vi "Lab Panel V4.86.vi"() -> ()   [LabVIEW 2013] (continued)
                  tunnel: w5309 -> [w5337 w5340]
                  tunnel: [w5337 w5339] -> w5307
                  frame False {
                  }
                  frame True {
                    n2929 = Multiply(x=w5341, y=w5340) -> (x*y=w5339:dbl)
                    n2930 = Multiply(x=w5341, y=w5343) -> (x*y=w5342:dbl)
                  }
                }
                n2931 = local read "SIG LAB05-1"() -> (w5328:T2)
                n2932 = Bundle By Name(cluster=w5328, "Tmp Live"=w5308, "Tmp Neut"=w5307) -> (w5327:T2)
                n2933 = local read "SIG LAB05-2"() -> (w5326:T2)
                n2934 = Bundle By Name(cluster=w5326, "Tmp Live"=w5304, "Tmp Neut"=w5303) -> (w5325:T2)
                n2935 = local write "SIG LAB05-1"(w5327) -> ()
                n2936 = local write "SIG LAB05-2"(w5325) -> ()
              }
            }
          }
          frame #20 {
            # "write data to display panel"
            n2937 = global write "Global display 1.vi" "TEST 5-2"(w5380) -> ()
            n2938 = global write "Global display 1.vi" "TEST 4-2"(w5382) -> ()
            n2939 = global write "Global display 1.vi" "TEST 1-2"(w5388) -> ()
            n2940 = global write "Global display 1.vi" "TEST 3-1"(w5385) -> ()
            n2941 = global write "Global display 1.vi" "TEST 5-1"(w5381) -> ()
            n2942 = global write "Global display 1.vi" "TEST 1-1"(w5389) -> ()
            n2943 = global write "Global display 1.vi" "TEST 3-2"(w5384) -> ()
            n2944 = global write "Global display 1.vi" "TEST 4-1"(w5383) -> ()
            n2945 = global write "Global display 1.vi" "TEST 2-2"(w5386) -> ()
            n2946 = global write "Global display 1.vi" "TEST 2-1"(w5387) -> ()
            n2947 = global read "Global display 3.vi" "log 1-1"() -> (→"LOG LAB01-1":string)
            n2948 = global read "Global display 3.vi" "log 3-1"() -> (→"LOG LAB03-1":string)
            n2949 = global read "Global display 3.vi" "log 1-2"() -> (→"LOG LAB01-2":string)
            n2950 = property on="Tab Control 2" class="TabCtl (strict)"() -> ("Pages"=w5379:refnum<vi>[])  [unwired: 2 in, 2 out]
            n2951 = global read "Global display 3.vi" "log 2-1"() -> (→"LOG LAB02-1":string)
            n2952 = global read "Global display 3.vi" "log 2-2"() -> (→"LOG LAB02-2":string)
            n2953 = global read "Global display 3.vi" "log 4-2"() -> (→"LOG LAB04-2":string)
            n2954 = global read "Global display 3.vi" "log 5-2"() -> (→"LOG LAB05-2":string)
            n2955 = global read "Global display 3.vi" "log 5-1"() -> (→"LOG LAB05-1":string)
            n2956 = global read "Global display 3.vi" "log 4-1"() -> (→"LOG LAB04-1":string)
            n2957 = global read "Global display 3.vi" "log 3-2"() -> (→"LOG LAB03-2":string)
            n2958 = Index Array(array=w5379, index=9) -> (element=w5377:refnum<vi>)
            n2959 = property class="Page"(reference=w5377) -> ("PageVis"=w5376:bool)  [unwired: 1 in, 2 out]
            n2960 = global write "Global display 3.vi" "admin"(w5376) -> ()
            n2961 = local read "O/I  LAB05-2"() -> (w5430:bool)
            n2962 = local read "O/I  LAB05-1"() -> (w5431:bool)
            n2963 = local read "O/I  LAB03-2"() -> (w5434:bool)
            n2964 = local read "O/I  LAB04-2"() -> (w5432:bool)
            n2965 = local read "O/I  LAB04-1"() -> (w5433:bool)
            n2966 = local read "O/I  LAB03-1"() -> (w5435:bool)
            n2967 = local read "O/I  LAB01-2"() -> (w5438:bool)
            n2968 = local read "O/I  LAB01-1"() -> (w5439:bool)
            n2969 = local read "O/I  LAB02-1"() -> (w5437:bool)
            n2970 = local read "O/I  LAB02-2"() -> (w5436:bool)
            n2971 = global write "Global display 1.vi" "5-2 O/F"(w5430) -> ()
            n2972 = global write "Global display 1.vi" "5-1 O/F"(w5431) -> ()
            n2973 = global write "Global display 1.vi" "4-1 O/F"(w5433) -> ()
            n2974 = global write "Global display 1.vi" "4-2 O/F"(w5432) -> ()
            n2975 = global write "Global display 1.vi" "3-2 O/F"(w5434) -> ()
            n2976 = global write "Global display 1.vi" "3-1 O/F"(w5435) -> ()
            n2977 = global write "Global display 1.vi" "2-2 O/F"(w5436) -> ()
            n2978 = global write "Global display 1.vi" "2-1 O/F"(w5437) -> ()
            n2979 = global write "Global display 1.vi" "1-2 O/F"(w5438) -> ()
            n2980 = global write "Global display 1.vi" "1-1 O/F"(w5439) -> ()
            n2981 = local read "TEMP START LAB02-2"() -> (w5362:cluster{"TL":dbl, "TN":dbl})
            n2982 = local read "run lab05-2"() -> (w5420:bool)
            n2983 = local read "TEMP START LAB01-2"() -> (w5364:cluster{"TL":dbl, "TN":dbl})
            n2984 = local read "TEMP START LAB02-1"() -> (w5363:cluster{"TL":dbl, "TN":dbl})
            n2985 = local read "TEMP START LAB04-1"() -> (w5359:cluster{"TL":dbl, "TN":dbl})
            n2986 = local read "TEMP START LAB04-2"() -> (w5358:cluster{"TL":dbl, "TN":dbl})
            n2987 = local read "run lab04-1"() -> (w5423:bool)
            n2988 = local read "run lab04-2"() -> (w5422:bool)
            n2989 = local read "run lab05-1"() -> (w5421:bool)
            n2990 = local read "TEMP START LAB01-1"() -> (w5365:cluster{"TL":dbl, "TN":dbl})
            n2991 = local read "TEMP START LAB05-2"() -> (w5356:cluster{"TL":dbl, "TN":dbl})
            n2992 = local read "TEMP START LAB05-1"() -> (w5357:cluster{"TL":dbl, "TN":dbl})
            n2993 = local read "run lab03-2"() -> (w5424:bool)
            n2994 = local read "TEMP START LAB03-2"() -> (w5360:cluster{"TL":dbl, "TN":dbl})
            n2995 = local read "TEMP START LAB03-1"() -> (w5361:cluster{"TL":dbl, "TN":dbl})
            n2996 = local read "run lab02-1"() -> (w5427:bool)
            n2997 = local read "run lab03-1"() -> (w5425:bool)
            n2998 = local read "run lab01-2"() -> (w5428:bool)
            n2999 = local read "run lab02-2"() -> (w5426:bool)
            n3000 = local read "run lab01-1"() -> (w5429:bool)
            n3001 = global write "Global display 1.vi" "5-2 R/S"(w5420) -> ()
            n3002 = global write "Global display 1.vi" "5-1 R/S"(w5421) -> ()
            n3003 = global write "Global display 1.vi" "4-2 R/S"(w5422) -> ()
            n3004 = global write "Global display 1.vi" "4-1 R/S"(w5423) -> ()
            n3005 = global write "Global display 1.vi" "3-2 R/S"(w5424) -> ()
            n3006 = global write "Global display 1.vi" "1-2 R/S"(w5428) -> ()
            n3007 = global write "Global display 1.vi" "2-1 R/S"(w5427) -> ()
            n3008 = global write "Global display 1.vi" "3-1 R/S"(w5425) -> ()
            n3009 = global write "Global display 1.vi" "2-2 R/S"(w5426) -> ()
            n3010 = global write "Global display 1.vi" "1-1 R/S"(w5429) -> ()
            n3011 = global write "Global display 3.vi" "TEMP ST 05-2"(w5356) -> ()
            n3012 = global write "Global display 3.vi" "TEMP ST 05-1"(w5357) -> ()
            n3013 = global write "Global display 3.vi" "TEMP ST 03-2"(w5360) -> ()
            n3014 = global write "Global display 3.vi" "TEMP ST 04-2"(w5358) -> ()
            n3015 = global write "Global display 3.vi" "TEMP ST 01-1"(w5365) -> ()
            n3016 = global write "Global display 3.vi" "TEMP ST 01-2"(w5364) -> ()
            n3017 = global write "Global display 3.vi" "TEMP ST 04-1"(w5359) -> ()
            n3018 = global write "Global display 3.vi" "TEMP ST 02-1"(w5363) -> ()
            n3019 = global write "Global display 3.vi" "TEMP ST 02-2"(w5362) -> ()
            n3020 = global write "Global display 3.vi" "TEMP ST 03-1"(w5361) -> ()
            n3021 = local read "DISP LAB04-2"() -> (w5412:T4)
            n3022 = local read "DISP LAB05-1"() -> (w5411:T4)
            n3023 = local read "DISP LAB04-1"() -> (w5413:T4)
            n3024 = local read "DISP LAB05-2"() -> (w5410:T4)
            n3025 = local read "DISP LAB03-1"() -> (w5415:T4)
            n3026 = local read "DISP LAB03-2"() -> (w5414:T4)
            n3027 = local read "DISP LAB01-2"() -> (w5418:T4)
            n3028 = local read "DISP LAB02-1"() -> (w5417:T4)
            n3029 = local read "DISP LAB02-2"() -> (w5416:T4)
            n3030 = local read "DISP LAB01-1"() -> (w5419:T4)
            n3031 = local read "TEMP RISE LAB05-1"() -> (w5347:cluster{"TL":dbl, "TN":dbl})
            n3032 = local read "TEMP RISE LAB05-2"() -> (w5346:cluster{"TL":dbl, "TN":dbl})
            n3033 = local read "TEMP RISE LAB04-2"() -> (w5348:cluster{"TL":dbl, "TN":dbl})
            n3034 = local read "TEMP RISE LAB04-1"() -> (w5349:cluster{"TL":dbl, "TN":dbl})
            n3035 = local read "TEMP RISE LAB03-2"() -> (w5350:cluster{"TL":dbl, "TN":dbl})
            n3036 = local read "TEMP RISE LAB03-1"() -> (w5351:cluster{"TL":dbl, "TN":dbl})
            n3037 = local read "TEMP RISE LAB01-2"() -> (w5354:cluster{"TL":dbl, "TN":dbl})
            n3038 = local read "TEMP RISE LAB02-2"() -> (w5352:cluster{"TL":dbl, "TN":dbl})
            n3039 = local read "TEMP RISE LAB01-1"() -> (w5355:cluster{"TL":dbl, "TN":dbl})
            n3040 = local read "TEMP RISE LAB02-1"() -> (w5353:cluster{"TL":dbl, "TN":dbl})
            n3041 = global write "Global display 2.vi" "DISP LAB05-1"(w5411) -> ()
            n3042 = global write "Global display 2.vi" "DISP LAB05-2"(w5410) -> ()
            n3043 = global write "Global display 2.vi" "DISP LAB04-2"(w5412) -> ()
            n3044 = global write "Global display 2.vi" "DISP LAB02-1"(w5417) -> ()
            n3045 = global write "Global display 2.vi" "DISP LAB02-2"(w5416) -> ()
            n3046 = global write "Global display 2.vi" "DISP LAB04-1"(w5413) -> ()
            n3047 = global write "Global display 2.vi" "DISP LAB01-2"(w5418) -> ()
            n3048 = global write "Global display 2.vi" "DISP LAB01-1"(w5419) -> ()
            n3049 = global write "Global display 2.vi" "DISP LAB03-1"(w5415) -> ()
            n3050 = global write "Global display 2.vi" "DISP LAB03-2"(w5414) -> ()
            n3051 = global write "Global display 3.vi" "TEMP RS 05-2"(w5346) -> ()
            n3052 = global write "Global display 3.vi" "TEMP RS 05-1"(w5347) -> ()
            n3053 = global write "Global display 3.vi" "TEMP RS 03-2"(w5350) -> ()
            n3054 = global write "Global display 3.vi" "TEMP RS 02-1"(w5353) -> ()
            n3055 = global write "Global display 3.vi" "TEMP RS 02-2"(w5352) -> ()
            n3056 = global write "Global display 3.vi" "TEMP RS 04-2"(w5348) -> ()
            n3057 = global write "Global display 3.vi" "TEMP RS 01-2"(w5354) -> ()
            n3058 = global write "Global display 3.vi" "TEMP RS 03-1"(w5351) -> ()
            n3059 = global write "Global display 3.vi" "TEMP RS 04-1"(w5349) -> ()
            n3060 = global write "Global display 3.vi" "TEMP RS 01-1"(w5355) -> ()
            n3061 = local read "SET LAB05-2"() -> (w5400:T5)
            n3062 = local read "SET LAB05-1"() -> (w5401:T5)
            n3063 = local read "SET LAB04-1"() -> (w5403:T5)
            n3064 = local read "SET LAB04-2"() -> (w5402:T5)
            n3065 = local read "SET LAB03-1"() -> (w5405:T5)
            n3066 = local read "SET LAB03-2"() -> (w5404:T5)
            n3067 = local read "SET LAB02-2"() -> (w5406:T5)
            n3068 = local read "SET LAB01-2"() -> (w5408:T5)
            n3069 = local read "SET LAB02-1"() -> (w5407:T5)
            n3070 = local read "SET LAB01-1"() -> (w5409:T5)
            n3071 = global write "Global display 2.vi" "SET LAB05-2"(w5400) -> ()
            n3072 = global write "Global display 2.vi" "SET LAB05-1"(w5401) -> ()
            n3073 = global write "Global display 2.vi" "SET LAB04-1"(w5403) -> ()
            n3074 = global write "Global display 2.vi" "SET LAB04-2"(w5402) -> ()
            n3075 = global write "Global display 2.vi" "SET LAB03-2"(w5404) -> ()
            n3076 = global write "Global display 2.vi" "SET LAB02-2"(w5406) -> ()
            n3077 = global write "Global display 2.vi" "SET LAB03-1"(w5405) -> ()
            n3078 = global write "Global display 2.vi" "SET LAB01-2"(w5408) -> ()
            n3079 = global write "Global display 2.vi" "SET LAB01-1"(w5409) -> ()
            n3080 = global write "Global display 2.vi" "SET LAB02-1"(w5407) -> ()
            n3081 = local read "RESULT LAB01-1"() -> (w5399:bool)
            n3082 = local read "RESULT LAB03-2"() -> (w5394:bool)
            n3083 = local read "RESULT LAB04-1"() -> (w5393:bool)
            n3084 = local read "RESULT LAB04-2"() -> (w5392:bool)
            n3085 = local read "RESULT LAB02-2"() -> (w5396:bool)
            n3086 = local read "RESULT LAB01-2"() -> (w5398:bool)
            n3087 = local read "RESULT LAB02-1"() -> (w5397:bool)
            n3088 = local read "RESULT LAB03-1"() -> (w5395:bool)
            n3089 = local read "RESULT LAB05-1"() -> (w5391:bool)
            n3090 = local read "RESULT LAB05-2"() -> (w5390:bool)
            n3091 = global write "Global display 2.vi" "RESULT LAB05-1"(w5391) -> ()
            n3092 = global write "Global display 2.vi" "RESULT LAB01-2"(w5398) -> ()
            n3093 = global write "Global display 2.vi" "RESULT LAB03-2"(w5394) -> ()
            n3094 = global write "Global display 2.vi" "RESULT LAB04-1"(w5393) -> ()
            n3095 = global write "Global display 2.vi" "RESULT LAB04-2"(w5392) -> ()
            n3096 = global write "Global display 2.vi" "RESULT LAB05-2"(w5390) -> ()
            n3097 = global write "Global display 2.vi" "RESULT LAB03-1"(w5395) -> ()
            n3098 = global write "Global display 2.vi" "RESULT LAB02-1"(w5397) -> ()
            n3099 = global write "Global display 2.vi" "RESULT LAB02-2"(w5396) -> ()
            n3100 = global write "Global display 2.vi" "RESULT LAB01-1"(w5399) -> ()
          }
          frame #21 {
            # "end main and display program"
            n3101 = Quit LabVIEW(quit? (T)="stop all") -> ()
            n3102 = global write "Global display 1.vi" "stop disp"("stop all") -> ()
          }
        }
        n3103 = node-c288() -> ()  [unwired: 1 in, 1 out]
        "loops" <- w292
      }
      n3104 = node-c288(w269) -> ()  [unwired: 1 out]
    }
  }
